vi "Configure Waveform Length.vi"(8 "error in (no error)":errorcluster, 9 "Set Points (1000)":i32=1000, 10 "Memory Name (0: Edit Memory)":i32(ring) items=["Edit Memory", "Edit Memory 1", "Edit Memory 2"], 11 "VISA resource name":refnum<visa-resource-name>) -> (0 "error out":errorcluster, 3 "VISA resource name out":refnum<visa-resource-name>)   [LabVIEW 2020, in "AWG.lvlib" / "Tektronix AFG 3000 Series.lvlib"]
doc: "Configures the number of data points for the waveform created in the edit memory.\n\n<B>Note:</B> \n\nThis VI is only applicable for AFG 3kC series."
uses:
  Tektronix AFG 3000 Series.lvlib
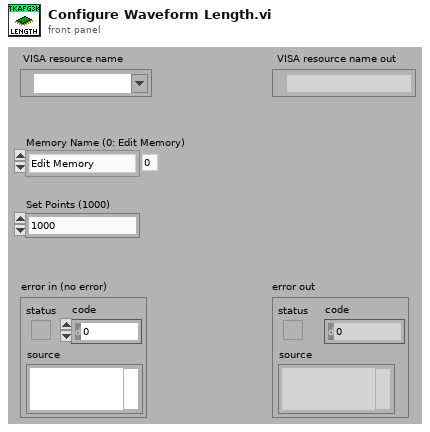
[diagram p1: front panel]
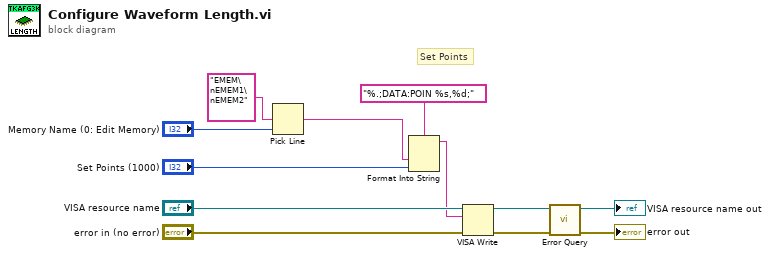
[diagram p0: block diagram]
diagram:
  # "Set Points"
  n1 = Pick Line(multi-line string="EMEM\nEMEM1\nEMEM2" ("string (\"\")"), line index="Memory Name (0: Edit Memory)") -> (output string=w9:string)  [unwired: 1 in]
  n2 = Format Into String(format string="%.;DATA:POIN %s,%d;", w9, "Set Points (1000)") -> (resulting string=w1:string)  [unwired: 2 in, 1 out]
  n3 = VISA Write(VISA resource name="VISA resource name", write buffer=w1, error in (no error)="error in (no error)") -> (VISA resource name out=w6:refnum<visa-resource-name>, error out=w4:errorcluster)  [unwired: 1 out]
  n4 = call "Error Query.vi"("error in (no error)"=w4, "VISA resource name"=w6) -> ("error out"=→"error out":errorcluster, "VISA resource name out"=→"VISA resource name out":refnum<visa-resource-name>)  [unwired: 6 in, 2 out]
